vi "currentHostPC.vi"() -> ()   [LabVIEW 2020]
panel:
  in  "stop":bool
  out "TIA":T1(graph)
  out "Currrent State TIA 3":dbl
  out "Currrent State TIA 2":dbl
  out "Currrent State TIA 1":dbl
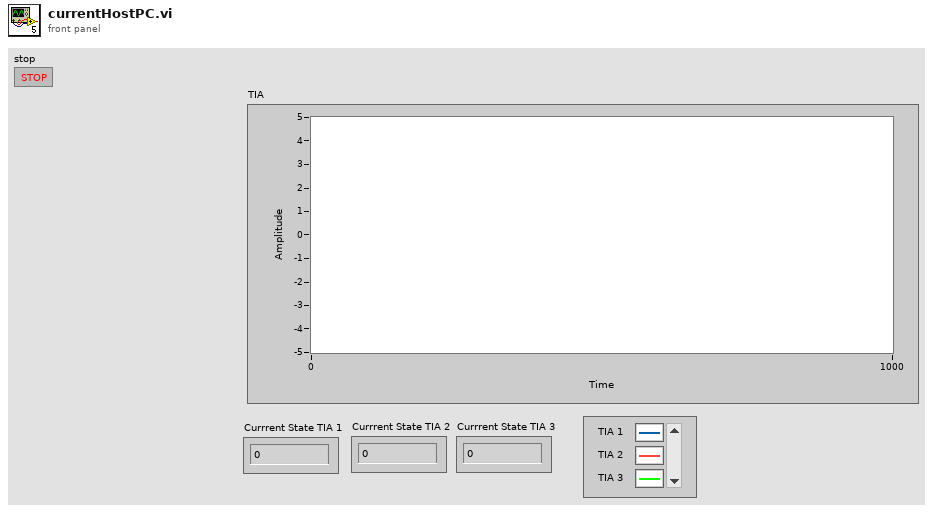
[diagram p1: front panel]
types:
  T1 = cluster{"Double":dbl, "Double":dbl, "Double":dbl}
  T2 = enum16{"open", "replace", "create", "open or create", "replace or create", "replace or create with confirmation"}
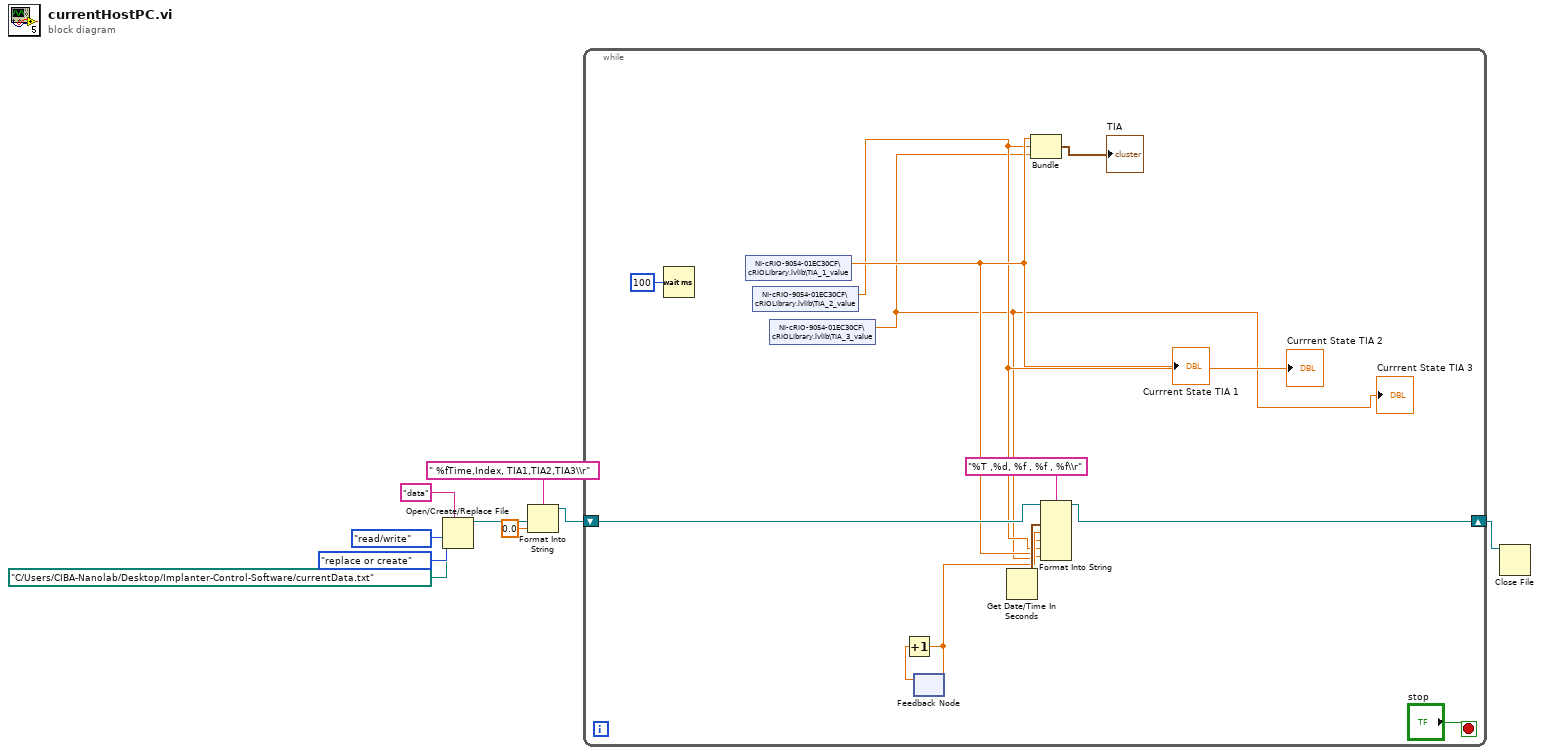
[diagram p0: block diagram]
diagram:
  n1 = Open/Create/Replace File(file path (use dialog)=path "C:/Users/CIBA-Nanolab/Desktop/Implanter-Control-Software/currentData.txt", prompt="data", operation (0:open)=T2."replace or create", access (0:read/write)=enum16{"read/write", "read-only", "write-only"}."read/write") -> (refnum out=w4:refnum<file>)  [unwired: 2 in, 2 out]
  n2 = Format Into String(format string=" %fTime,Index, TIA1,TIA2,TIA3\\r", initial string=w4, 0.0 ("input 1")) -> (resulting string=w3:refnum<file>)  [unwired: 1 in, 1 out]
  n3 = while {
    shift-right: [w18] -> w2
    shift-left: w3 -> [w19]
    stop <- "stop" stop-if-true
    n4 = Wait (ms)(milliseconds to wait=u32 100) -> ()  [unwired: 1 out]
    n5 = shared-variable "NI-cRIO-9054-01EC30CF\\cRIOLibrary.lvlib\\TIA_1_value"() -> (w12:dbl)  [unwired: 1 in, 1 out]
    "Currrent State TIA 1" <- w12
    n6 = shared-variable "NI-cRIO-9054-01EC30CF\\cRIOLibrary.lvlib\\TIA_2_value"() -> (w11:dbl)  [unwired: 1 in, 1 out]
    "Currrent State TIA 2" <- w11
    n7 = shared-variable "NI-cRIO-9054-01EC30CF\\cRIOLibrary.lvlib\\TIA_3_value"() -> (w10:dbl)  [unwired: 1 in, 1 out]
    "Currrent State TIA 3" <- w10
    n8 = feedback #1() -> (w14:dbl)  [unwired: 1 in]
    n9 = Increment(x=w14) -> (x+1=w13:dbl)
    n10 = feedback-in #1(w13) -> ()
    n11 = Get Date/Time In Seconds() -> (seconds since 1Jan1904=w17:timestamp)
    n12 = Bundle("Double"=w12, "Double"=w11, "Double"=w10) -> (→"TIA":T1)  [unwired: 1 in]
    n13 = Format Into String(format string="%T ,%d, %f , %f , %f\\r", initial string=w19, w17, w13, w12, w11, w10) -> (resulting string=w18:refnum<file>)  [unwired: 1 in, 1 out]
  }
  n14 = Close File(refnum=w2) -> ()  [unwired: 1 in, 2 out]
